vi "Get_HEATERS_Values_From_JSON.vi"(8 "Error In":errorcluster, 10 "utf-8 text":string="{\"status\": \"OK\", \"data\": [{\"control_algorithm_settings\": {\"proportional\": 0.0, \"integral\": 0.0, \"derivative\": 0}, \"name\": \"Heatswitch Still\", \"power\": 0.108, \"relay_mode\": 0, \"target_temperature_shown\": false, \"heater_nr\": 1, \"resistance\": 30.0, \"control_algorithm\": 1, \"max_power\": 0.11, \"pid_mode\": 0, \"active\": true, \"target_temperature\": 0.01, \"setpoint\": 0.01, \"relay_status\": 0}, {\"control_algorithm_settings\": {\"proportional\": 0.0, \"integral\": 0.0, \"derivative\": 0}, \"name\": \"Heatswitch MXC\", \"power\": 0.054, \"relay_mode\": 0, \"target_temperature_shown\": false, \"heater_nr\": 2, \"resistance\": 60.0, \"control_algorithm\": 1, \"max_power\": 0.056, \"pid_mode\": 0, \"active\": true, \"target_temperature\": 0.01, \"setpoint\": 0.01, \"relay_status\": 0}, {\"control_algorithm_settings\": {\"proportional\": 0.0, \"integral\": 0.0, \"derivative\": 0}, \"name\": \"Still-heater\", \"power\": 0.006, \"relay_mode\": 0, \"target_temperature_shown\": false, \"heater_nr\": 3, \"resistance\": 120, \"control_algorithm\": 1, \"max_power\": 1.0, \"pid_mode\": 0, \"active\": true, \"target_temperature\": 0.01, \"setpoint\": 0.01, \"relay_status\": 1}, {\"control_algorithm_settings\": {\"proportional\": 0.01, \"integral\": 100, \"derivative\": 0}, \"name\": \"MXC-heater\", \"power\": 0.004317939987440146, \"relay_mode\": 1, \"target_temperature_shown\": false, \"heater_nr\": 4, \"resistance\": 120, \"control_algorithm\": 1, \"max_power\": 0.004317939987440146, \"pid_mode\": 1, \"active\": false, \"target_temperature\": 0.01, \"setpoint\": 0.4, \"relay_status\": 1}], \"datetime\": \"2023-02-04T20:06:44.587060Z\"}") -> (0 "Error Out":errorcluster, 1 "value":T1)   [LabVIEW 2017]
panel:
  in  "path":string[](array[string])
  in  "Cluster":T1
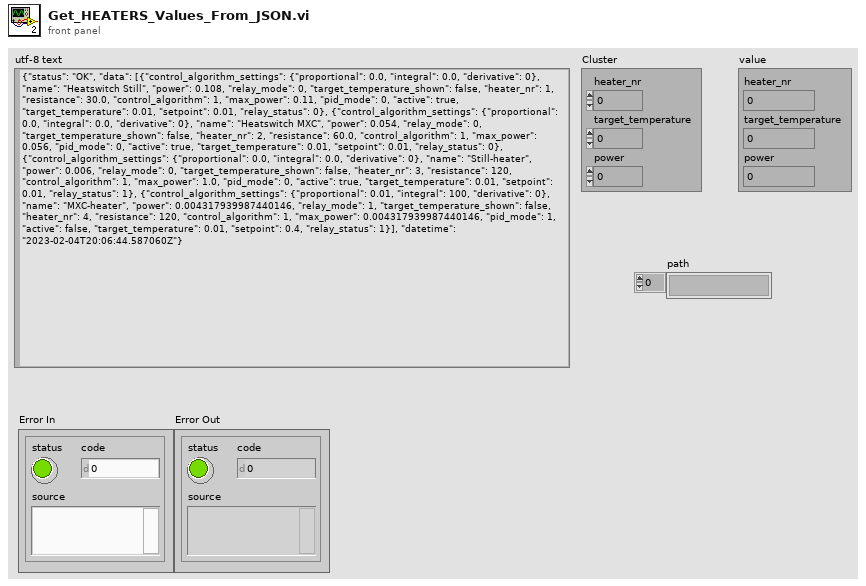
[diagram p1: front panel]
types:
  T1 = cluster{"heater_nr":i32, "target_temperature":dbl, "power":dbl}
  T2 = cluster{"id":i32, "name":string, "description":string}
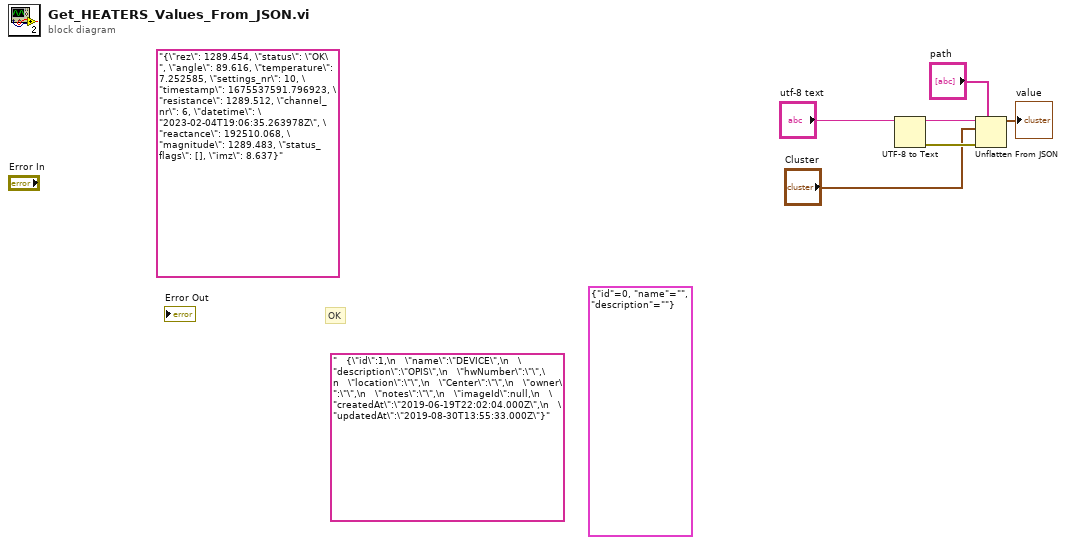
[diagram p0: block diagram]
diagram:
  (unwired) "{\"rez\": 1289.454, \"status\": \"OK\", \"angle\": 89.616, \"temperature\": 7.252585, \"settings_nr\": 10, \"timestamp\": 1675537591.796923, \"resistance\": 1289.512, \"channel_nr\": 6, \"datetime\": \"2023-02-04T19:06:35.263978Z\", \"reactance\": 192510.068, \"magnitude\": 1289.483, \"status_flags\": [], \"imz\": 8.637}" ("utf-8 text")
  (unwired) T2 {"id"=0, "name"="", "description"=""}
  (unwired) "   {\"id\":1,\n   \"name\":\"DEVICE\",\n   \"description\":\"OPIS\",\n   \"hwNumber\":\"\",\n   \"location\":\"\",\n   \"Center\":\"\",\n   \"owner\":\"\",\n   \"notes\":\"\",\n   \"imageId\":null,\n   \"createdAt\":\"2019-06-19T22:02:04.000Z\",\n   \"updatedAt\":\"2019-08-30T13:55:33.000Z\"}" ("utf-8 text")
  # "OK"
  n1 = UTF-8 to Text(11:"utf-8 text") -> (0:w6:errorcluster, 3:w3:string)  [unwired: 2 in]
  n2 = Unflatten From JSON(path="path", JSON string=w3, type and defaults="Cluster", error in (no error)=w6) -> (value=→"value":T1)  [unwired: 3 in, 1 out]
